vi "Voltage - Finite Input.vi"() -> ()   [LabVIEW 2017]
doc: "This example demonstrates how to acquire a single buffer of voltage measurements using a DAQmx device.\n\nFor instructions on how to connect your signals to the DAQ device, refer to your device documentation."
uses:
  <vilib>/Utility/error.llb/DialogType.ctl
  <vilib>/DAQmx/read.llb/DAQmx Read (Analog 1D Wfm NChan NSamp).vi
  <vilib>/DAQmx/create/channels.llb/DAQmx Create Channel (AI-Voltage-Basic).vi
  <vilib>/DAQmx/configure/timing.llb/DAQmx Timing (Sample Clock).vi
  <vilib>/DAQmx/configure/task.llb/DAQmx Configure Logging (TDMS).vi
  <vilib>/DAQmx/configure/trigger.llb/DAQmx Start Trigger (Digital Edge).vi
  <vilib>/DAQmx/configure/trigger.llb/DAQmx Start Trigger (Analog Edge).vi
  <vilib>/DAQmx/configure/trigger.llb/DAQmx Reference Trigger (Digital Edge).vi
  <vilib>/DAQmx/configure/trigger.llb/DAQmx Reference Trigger (Analog Edge).vi
  <vilib>/DAQmx/miscellaneous.llb/DAQmx Fill In Error Info.vi
  <resource>/objmgr/daqmx.rc
panel:
  in  "Trigger Type":T1(tab)
  in  "Digital Start Trigger Edge":i32(ring)=10280 caption="Edge" items=["Rising"=10280, "Falling"=10171]
  in  "Digital Start Trigger Source":tag="/Dev1/PFI0" caption="Source"
  in  "Digital Pause Trigger Pause When":i32(ring)=10192 caption="Pause When" items=["High"=10192, "Low"=10214]
  in  "Digital Pause Trigger Source":tag="/Dev1/PFI0" caption="Source"
  in  "Digital Reference Trigger Source":tag="/Dev1/PFI0" caption="Source"
  in  "Digital Reference Trigger Edge":i32(ring)=10280 caption="Edge" items=["Rising"=10280, "Falling"=10171]
  in  "Digital Reference Pretrigger Samples":u32 caption="Pretrigger Samples"
  in  "Analog Start Trigger Level":dbl caption="Level" format="%0.2f"
  in  "Analog Start Trigger Hysteresis":dbl caption="Hysteresis" format="%.2f"
  in  "Analog Start Trigger Slope":i32(ring)=10280 caption="Slope" items=["Rising"=10280, "Falling"=10171]
  in  "Analog Start Trigger Source":string="APFI0" caption="Source"
  in  "Analog Pause Trigger Source":string="APFI0" caption="Source"
  in  "Analog Pause Trigger Pause When":i32(ring)=10093 caption="Pause When" items=["Above Level"=10093, "Below Level"=10107]
  in  "Analog Pause Trigger Level":dbl caption="Level" format="%.2f"
  in  "Analog Reference Trigger Source":string="APFI0" caption="Source"
  in  "Analog Reference Trigger Level":dbl caption="Level" format="%.2f"
  in  "Analog Reference Trigger Slope":i32(ring)=10280 caption="Slope" items=["Rising"=10280, "Falling"=10171]
  in  "Analog Reference Pretrigger Samples":u32 caption="Pretrigger Samples"
  out "Waveform Graph":waveform(dbl)[](graph)
  in  "TDMS File Path":path
  in  "Number of Samples":i32=100
  in  "Sample Rate":dbl=1000.0
  in  "Sample Clock Source":tag="OnboardClock"
  in  "Terminal Configuration":i32(ring)=-1 items=["default"=-1, "RSE"=10083, "NRSE"=10078, "Differential"=10106, "Pseudodifferential"=12529]
  in  "Max Voltage":dbl=5.0
  in  "Min Voltage":dbl=-5.0
  in  "Physical Channel":tag="Dev1/ai0"
  out "Actual Sample Rate":dbl=1000.0 format="%0.2f"
  in  "Logging Mode":i32(ring)=10231 items=["Off"=10231, "Log and Read"=15842]
  # "Channel Settings"
  # "Acquired Data"
  # "Timing Settings"
  # "Trigger Settings"
  # "Logging Settings"
  # "To enable triggers, select a tab above, and configure the settings.\n\nNot all hardware supports all trigger types. Refer to your device documentation for more information."
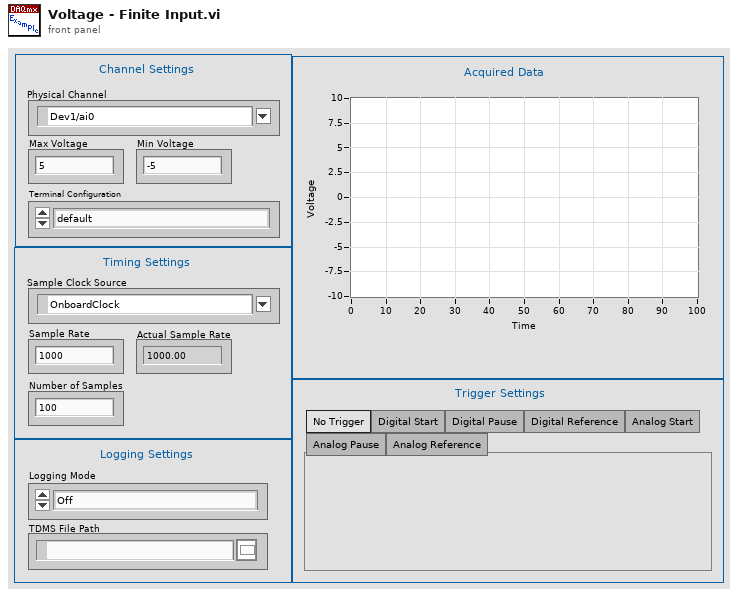
[diagram p1: front panel]
types:
  T1 = enum32{"No Trigger", "Digital Start", "Digital Pause", "Digital Reference", "Analog Start", "Analog Pause", "Analog Reference"}
  T2 = typedef "DialogType.ctl" = u16
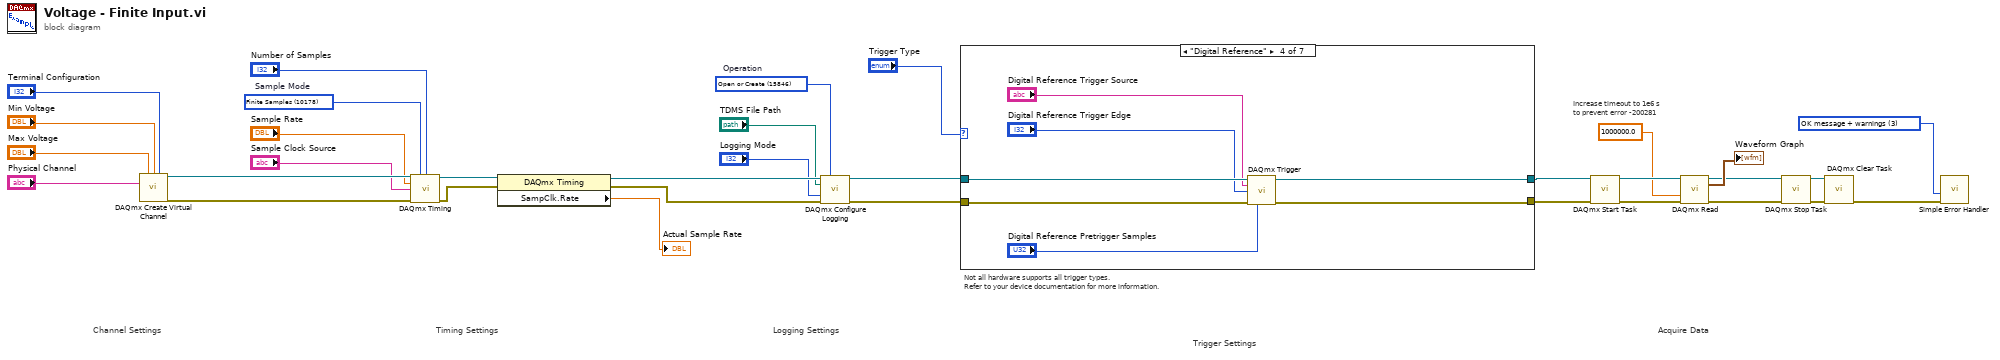
[diagram p0: block diagram]
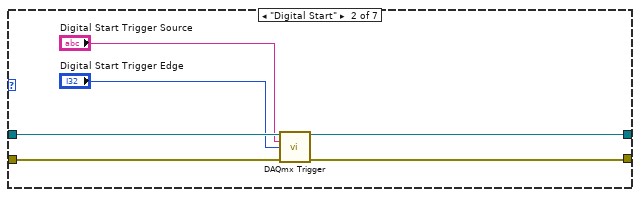
[diagram p3: hidden frame]
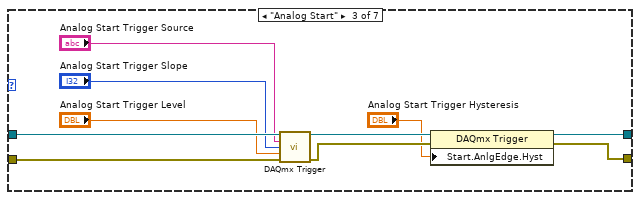
[diagram p4: hidden frame]
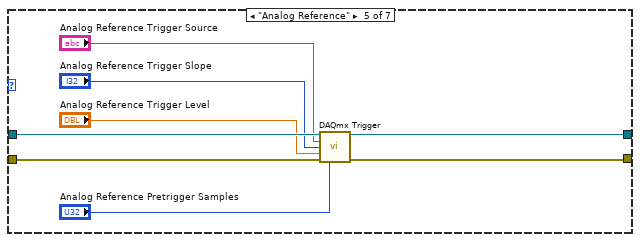
[diagram p5: hidden frame]
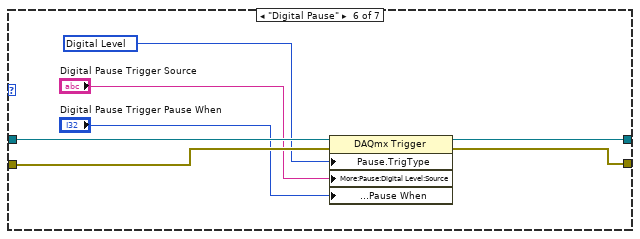
[diagram p6: hidden frame]
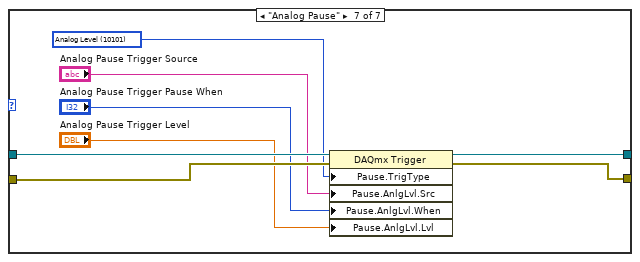
[diagram p7: hidden frame]
diagram:
  w7 = T2 3 items=["no dialog", "OK message", "continue or stop message", "OK message + warnings", "continue/stop + warnings"] ("type of dialog (OK msg:1)")
  w26 = 15846 items=["Open"=10437, "Open or Create"=15846, "Create or Replace"=15847, "Create"=15848]  # Operation
  w31 = 10178 items=["Finite Samples"=10178, "Continuous Samples"=10123, "Hardware Timed Single Point"=12522]  # Sample Mode
  # "Increase timeout to 1e6 s\nto prevent error -200281"
  # "Not all hardware supports all trigger types.\nRefer to your device documentation for more information."
  # "Trigger Settings"
  # "Acquire Data"
  # "Timing Settings"
  # "Channel Settings"
  # "Logging Settings"
  n1 = call-poly <vilib>:"DAQmx Create Virtual Channel.vi"("maximum value"="Max Voltage", "minimum value"="Min Voltage", "input terminal configuration"="Terminal Configuration", "physical channels"="Physical Channel") -> ("task out"=w29:refnum<k21>, "error out"=w30:errorcluster)  [unwired: 10 in]
  n2 = call-poly <vilib>:"DAQmx Timing.vi"("task/channels in"=w29, "sample mode"=w31, "samples per channel"="Number of Samples", "rate"="Sample Rate", "source"="Sample Clock Source", "error in"=w30) -> ("task out"=w33:refnum<k21>, "error out"=w32:errorcluster)  [unwired: 8 in]
  n3 = property class="DAQmx Timing"(reference=w33, error in=w32) -> (reference out=w28:refnum<k21>, error out=w27:errorcluster, "SampClk.Rate"=→"Actual Sample Rate":dbl)
  n4 = call-poly <vilib>:"DAQmx Configure Logging.vi"("task/channels in"=w28, "operation"=w26, "file path"="TDMS File Path", "logging mode"="Logging Mode", "error in"=w27) -> ("task out"=w5:refnum<k21>, "error out"=w4:errorcluster)  [unwired: 9 in]
  n5 = case shown="\"Digital Reference\"" "Trigger Type" {
    tunnel: w5 -> [w35 w41 w51 w58 w66 w73 w81]
    tunnel: w4 -> [w34 w40 w50 w57 w65 w70 w78]
    tunnel: [w35 w39 w48 w56 w64 w72 w80] -> w3
    tunnel: [w34 w38 w47 w55 w63 w71 w79] -> w2
    frame "No Trigger", Default {
    }
    frame "Digital Start" {
      n6 = call-poly <vilib>:"DAQmx Trigger.vi"("task/channels in"=w41, "source"="Digital Start Trigger Source", "edge"="Digital Start Trigger Edge", "error in"=w40) -> ("task out"=w39:refnum<k21>, "error out"=w38:errorcluster)  [unwired: 10 in]
    }
    frame "Analog Start" {
      n7 = call-poly <vilib>:"DAQmx Trigger.vi"("task/channels in"=w51, "source"="Analog Start Trigger Source", "slope"="Analog Start Trigger Slope", "level"="Analog Start Trigger Level", "error in"=w50) -> ("task out"=w46:refnum<k21>, "error out"=w45:errorcluster)  [unwired: 9 in]
      n8 = property class="DAQmx Trigger"(reference=w46, error in=w45, "Start.AnlgEdge.Hyst"="Analog Start Trigger Hysteresis") -> (reference out=w48:refnum<k21>, error out=w47:errorcluster)
    }
    frame "Digital Reference" {
      n9 = call-poly <vilib>:"DAQmx Trigger.vi"("task/channels in"=w58, "source"="Digital Reference Trigger Source", "edge"="Digital Reference Trigger Edge", "error in"=w57, "pretrigger samples per channel"="Digital Reference Pretrigger Samples") -> ("task out"=w56:refnum<k21>, "error out"=w55:errorcluster)  [unwired: 9 in]
    }
    frame "Analog Reference" {
      n10 = call-poly <vilib>:"DAQmx Trigger.vi"("task/channels in"=w66, "source"="Analog Reference Trigger Source", "slope"="Analog Reference Trigger Slope", "level"="Analog Reference Trigger Level", "error in"=w65, "pretrigger samples per channel"="Analog Reference Pretrigger Samples") -> ("task out"=w64:refnum<k21>, "error out"=w63:errorcluster)  [unwired: 8 in]
    }
    frame "Digital Pause" {
      w69 = 10152 items=["Analog Level"=10101, "Analog Window"=10103, "Digital Level"=10152, "Digital Pattern"=10398, "None"=10230] ("Pause.TrigType")
      n11 = property class="DAQmx Trigger"(reference=w73, error in=w70, "Pause.TrigType"=w69, "More:Pause:Digital Level:Source"="Digital Pause Trigger Source", "More:Pause:Digital Level:Pause When"="Digital Pause Trigger Pause When") -> (reference out=w72:refnum<k21>, error out=w71:errorcluster)
    }
    frame "Analog Pause" {
      w77 = 10101 items=["Analog Level"=10101, "Analog Window"=10103, "Digital Level"=10152, "Digital Pattern"=10398, "None"=10230] ("Pause.TrigType")
      n12 = property class="DAQmx Trigger"(reference=w81, error in=w78, "Pause.TrigType"=w77, "Pause.AnlgLvl.Src"="Analog Pause Trigger Source", "Pause.AnlgLvl.When"="Analog Pause Trigger Pause When", "Pause.AnlgLvl.Lvl"="Analog Pause Trigger Level") -> (reference out=w80:refnum<k21>, error out=w79:errorcluster)
    }
  }
  n13 = call <vilib>:"DAQmx Start Task.vi"("task/channels in"=w3, "error in"=w2) -> ("task out"=w25:refnum<k21>, "error out"=w24:errorcluster)  [unwired: 12 in]
  n14 = call-poly <vilib>:"DAQmx Read.vi"("task/channels in"=w25, "timeout"=1000000.0, "error in"=w24) -> ("task out"=w9:refnum<k21>, "data"=→"Waveform Graph":waveform(dbl)[], "error out"=w8:errorcluster)  [unwired: 10 in]
  n15 = call <vilib>:"DAQmx Stop Task.vi"("task/channels in"=w9, "error in"=w8) -> ("task out"=w11:refnum<k21>, "error out"=w10:errorcluster)  [unwired: 12 in]
  n16 = call <vilib>:"DAQmx Clear Task.vi"("task in"=w11, "error in"=w10) -> ("error out"=w23:errorcluster)  [unwired: 13 in]
  n17 = call <vilib>:"Simple Error Handler.vi"("type of dialog (OK msg:1)"=w7, "error in (no error)"=w23) -> ()  [unwired: 3 in, 5 out]
